vi "expand.vi"(8 "error in (no error)":errorcluster, 9 "expansion_y":u32, 10 "expansion_x":u32, 11 "Structure in":refnum<class "Structure.lvclass">) -> (0 "error out":errorcluster, 3 "Structure out":refnum<class "Structure.lvclass">)   [LabVIEW 2023, in "TLC_Scripto.lvlib" / "Structure.lvclass"]
uses:
  Structure.lvclass
  Structure.lvclass/Structure.ctl
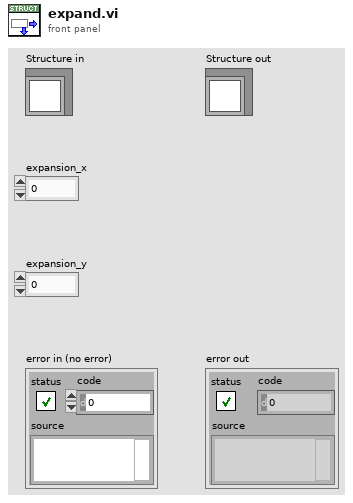
[diagram p1: front panel]
types:
  T1 = typedef "LVBoundsTypeDef.ctl" = cluster{"Width":u32, "Height":u32}
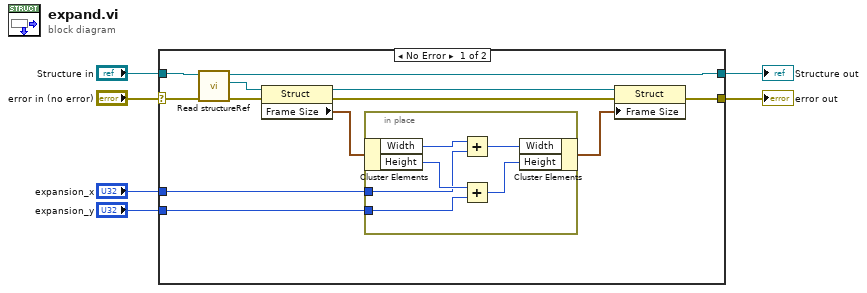
[diagram p0: block diagram]
diagram:
  n1 = case shown="No Error" "error in (no error)" {
    selector: "error in (no error)" -> [w18 w26]
    tunnel: [w12 w26] -> w5
    tunnel: [w10 w25] -> w3
    tunnel: "Structure in" -> [w9 w25]
    tunnel: "expansion_x" -> [w7 _]
    tunnel: "expansion_y" -> [w8 _]
    frame No Error {
      n2 = call "Read structureRef.vi"("error in (no error)"=w18, "Structure In"=w9) -> ("error out"=w13:errorcluster, "nodeRef"=w17:refnum<vi>, "Structure Out"=w10:refnum<class "Structure.lvclass">)  [unwired: 7 in]
      n3 = property class="Struct"(reference=w17, error in=w13) -> (reference out=w15:refnum<vi>, error out=w11:errorcluster, "Frame Size"=w14:T1)
      n4 = in-place {
        in-place-border: w8 -> [w21]
        in-place-border: w7 -> [w19]
        n5 = in-place-cluster #1(w14) -> ("Width"=w24:u32, "Height"=w22:u32)
        n6 = Add(x=w24, y=w19) -> (x+y=w23:u32)
        n7 = Add(x=w22, y=w21) -> (x+y=w20:u32)
        n8 = in-place-cluster #1("Width"=w23, "Height"=w20) -> (w16:T1)
      }
      n9 = property class="Struct"(reference=w15, error in=w11, "Frame Size"=w16) -> (error out=w12:errorcluster)  [unwired: 1 out]
    }
    frame Error {
    }
  }
  "error out" <- w5
  "Structure out" <- w3
